vi "Averaging Smooth.vi"(6 "Input":dbl, 8 "# of Samples to Average":dbl) -> (0 "array w/ subset deleted":dbl[](array[numeric]), 2 "Output":dbl)   [LabVIEW 2015]
doc: "This VI smooths the output by average a given number of input samples."
uses:
  <vilib>/Analysis/baseanly.llb/Mean (DBL).vi
  <vilib>/Analysis/NI_AALBase.lvlib
panel:
  # "Inputs"
  # "Process Variables"
  # "Outputs"
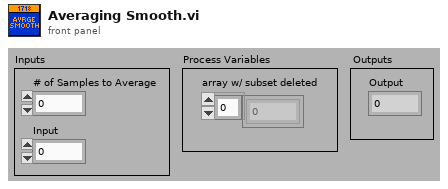
[diagram p1: front panel]
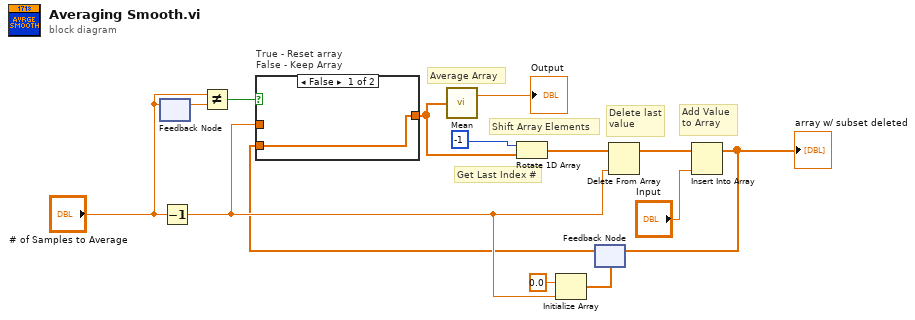
[diagram p0: block diagram]
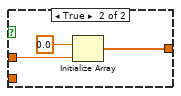
[diagram p2: hidden frame]
diagram:
  # "Delete last\nvalue"
  # "Shift Array Elements"
  # "Get Last Index #"
  # "Add Value\nto Array"
  # "Average Array"
  n1 = feedback #1() -> (w9:dbl)  [unwired: 1 in]
  n2 = feedback-in #1("# of Samples to Average") -> ()
  n3 = Decrement(x="# of Samples to Average") -> (x-1=w4:dbl)
  n4 = Not Equal?(x="# of Samples to Average", y=w9) -> (x != y?=w8:bool)
  n5 = Initialize Array(0.0 ("element"), w4) -> (w5:dbl[])
  n6 = feedback #2(w5) -> (w2:dbl[])
  n7 = case "True - Reset array\nFalse - Keep Array" shown="False" w8 {
    tunnel: w4 -> [_ w18]
    tunnel: [w15 w17] -> w7
    tunnel: w2 -> [w15 _]
    frame False {
    }
    frame True {
      n8 = Initialize Array(0.0 ("# of Samples\nto Average"), w18) -> (w17:dbl[])
    }
  }
  n9 = call-poly <vilib>:"Mean.vi"("X"=w7) -> ("mean"=→"Output":dbl)  [unwired: 1 out]
  n10 = Rotate 1D Array(1:w7, 2:-1 ("n")) -> (0:w12:dbl[])
  n11 = Delete From Array(array=w12, index=w4) -> (array with subset deleted=w11:dbl[])  [unwired: 1 in, 1 out]
  n12 = Insert Into Array(array=w11, new element="Input") -> (w10:dbl[])  [unwired: 1 in]
  "array w/ subset deleted" <- w10
  n13 = feedback-in #2(w10) -> ()
